vi "Exp_Setup_Control.vi"(2 "Source Control?":bool) -> ()   [LabVIEW 2022 SP3]
uses:
  ADAM Controls/Channel_State.ctl
  Channel_State_Control.ctl
  Anemometry/Anemometry Sub Vis/Globals/Trav_pos_global.vi
  Anemometry/Anemometry Sub Vis/Globals/Preference_global.vi
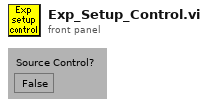
[diagram p1: front panel]
types:
  T1 = typedef "GMU Gas Line Name.ctl" = enum16{"GMU1 Source", "GMU2 Source", "GMU2 Calib", "CPP GRC-A", "CPP GRC-B"}
  T2 = typedef "Channel_State.ctl" = enum16{"On", "Off", "Always On", "Always Off"}
  T3 = typedef "Channel_State_Control.ctl" = enum16{"Channel Name", "Channel Name Starts with", "Main Address"}
  T4 = typedef "Ch_description_ADAM.ctl" = cluster{"Ch Name":string, "Type":T5, "Function":T6, "Ch State":T2, "Calibration type":T7, "A":dbl, "B":dbl, "C":dbl, "D":dbl, "Comments":string, "Address":T8, "String":string, "Duty":u16}
  T5 = typedef "Module_type_ADAM.ctl" = string
  T6 = typedef "Function_ADAM.ctl" = enum16{"Analogue Input", "Digital Input", "Event counter", "Event rate", "Analogue Output", "Digital Output", "Relay Output"}
  T7 = typedef "Calib_type_ADAM.ctl" = string
  T8 = typedef "Address.ctl" = cluster{"Main":i32, "Ch.":i32, "Sub":i32, "Port Name":string}
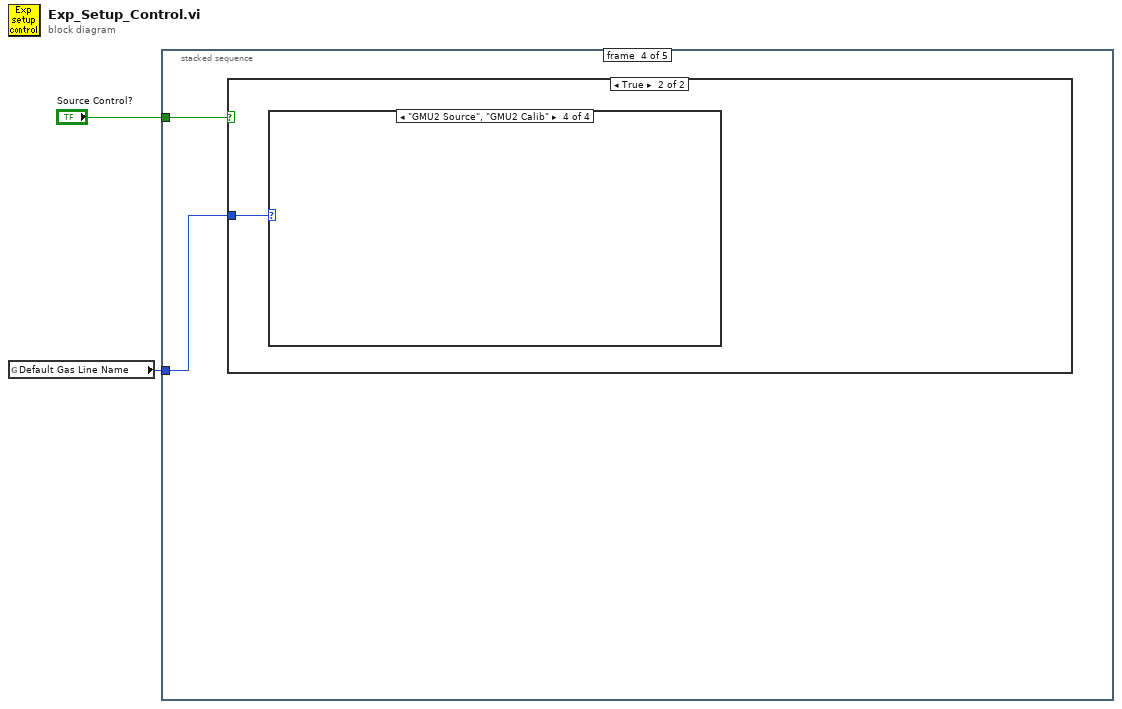
[diagram p0: block diagram]
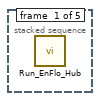
[diagram p2: hidden frame]
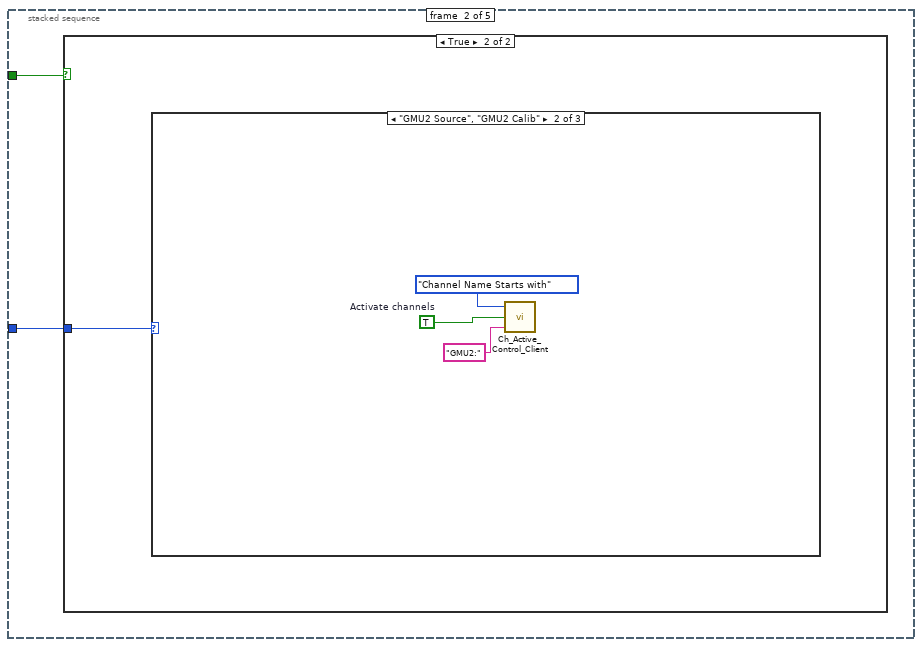
[diagram p3: hidden frame]
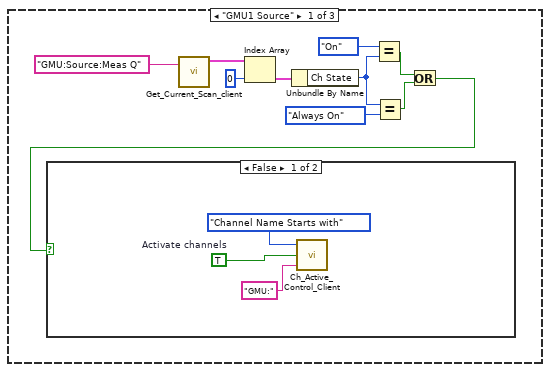
[diagram p5: hidden frame]
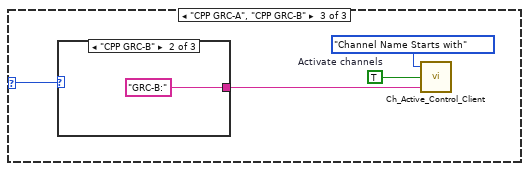
[diagram p7: hidden frame]
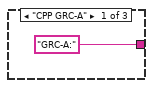
[diagram p8: hidden frame]
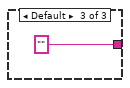
[diagram p9: hidden frame]
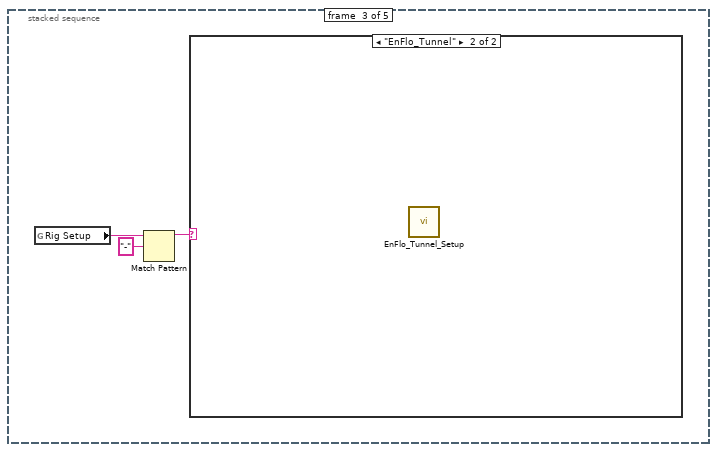
[diagram p10: hidden frame]
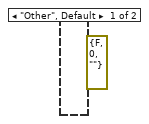
[diagram p11: hidden frame]
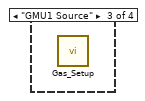
[diagram p15: hidden frame]
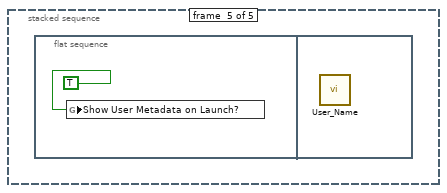
[diagram p16: hidden frame]
diagram:
  n1 = global read "Trav_pos_global.vi" "Default Gas Line Name"() -> (w1:T1)
  n2 = stacked-sequence {
    tunnel: "Source Control?" -> [_ w4 _ w33 _]
    tunnel: w1 -> [_ w3 _ w32 _]
    frame #0 {
      n3 = call "Run_EnFlo_Hub.vi"() -> ()  [unwired: 1 in, 7 out]
    }
    frame #1 {
      n4 = case shown="True" w4 {
        tunnel: w3 -> [_ w5]
        frame False {
        }
        frame True {
          n5 = case shown="\"GMU2 Source\", \"GMU2 Calib\"" w5 {
            selector: w5 -> [_ _ w23]
            frame "GMU1 Source" {
              n6 = call "Get_Current_Scan_client.vi"("singleChannel"="GMU:Source:Meas Q") -> ("Ch Description Array"=w15:T4[])  [unwired: 1 in, 3 out]
              n7 = Index Array(array=w15, index=0 ("Index")) -> (element=w13:T4)
              n8 = Unbundle By Name(w13) -> ("Ch State"=w11:T2)
              n9 = Equal?(x=Channel_State."On" ("Channel State"), y=w11) -> (x = y?=w8:bool)
              n10 = Equal?(x=w11, y=Channel_State."Always On" ("Channel State")) -> (x = y?=w9:bool)
              n11 = Or(x=w8, y=w9) -> (x .or. y?=w7:bool)
              n12 = case shown="False" w7 {
                frame False {
                  w16 = TRUE  # Activate channels
                  n13 = call "Ch_Active_Control_Client.vi"("Match"="GMU:", "Activate Channels?"=w16, "Control on"=Channel_State_Control."Channel Name Starts with") -> ()  [unwired: 2 out]
                }
                frame True {
                }
              }
            }
            frame "GMU2 Source", "GMU2 Calib" {
              w19 = TRUE  # Activate channels
              n14 = call "Ch_Active_Control_Client.vi"("Match"="GMU2:", "Activate Channels?"=w19, "Control on"=Channel_State_Control."Channel Name Starts with") -> ()  [unwired: 2 out]
            }
            frame "CPP GRC-A", "CPP GRC-B" {
              w25 = TRUE  # Activate channels
              n15 = case shown="\"CPP GRC-B\"" w23 {
                tunnel: ["GRC-A:" ("Match") "GRC-B:" ("Match") "" ("Match")] -> w22
                frame "CPP GRC-A" {
                }
                frame "CPP GRC-B" {
                }
                frame Default {
                }
              }
              n16 = call "Ch_Active_Control_Client.vi"("Match"=w22, "Activate Channels?"=w25, "Control on"=Channel_State_Control."Channel Name Starts with") -> ()  [unwired: 2 out]
            }
          }
        }
      }
    }
    frame #2 {
      n17 = global read "Preference_global.vi" "Rig Setup"() -> (w30:string)
      n18 = Match Pattern(string=w30, regular expression="-") -> (before substring=w29:string)  [unwired: 4 out]
      n19 = case shown="\"EnFlo_Tunnel\"" w29 {
        frame "Other", Default {
          (unwired) errorcluster {"status"=FALSE, "code"=0, "source"=""} ("error out")
        }
        frame "EnFlo_Tunnel" {
          n20 = call "EnFlo_Tunnel_Setup.vi"() -> ()  [unwired: 9 out]
        }
      }
    }
    frame #3 {
      n21 = case shown="True" w33 {
        tunnel: w32 -> [_ w34]
        frame False {
        }
        frame True {
          n22 = case shown="\"GMU2 Source\", \"GMU2 Calib\"" w34 {
            frame "CPP GRC-B" {
            }
            frame "CPP GRC-A" {
            }
            frame "GMU1 Source" {
              n23 = call "Gas_Setup.vi"() -> ()  [unwired: 9 out]
            }
            frame "GMU2 Source", "GMU2 Calib" {
            }
          }
        }
      }
    }
    frame #4 {
      n24 = flat-sequence {
        frame #0 {
          n25 = global write "Trav_pos_global.vi" "Show User Metadata on Launch?"(TRUE) -> ()
        }
        frame #1 {
          n26 = call "User_Name.vi"() -> ()  [unwired: 1 out]
        }
      }
    }
  }
